vi "FunctDataMgr.Update Meas Data.vi"(8 "error in (no error)":errorcluster, 10 "Data.Meas":T1[](array[typedef]) {"Status" items=["LOG", "PASS", "FAIL", "ERROR"]}, 11 "FunctDataMgr in":refnum<class "FunctDataMgr.lvclass">) -> (0 "error out":errorcluster, 3 "FunctDataMgr out":refnum<class "FunctDataMgr.lvclass">)   [LabVIEW 2024, in "FunctDataMgr.lvclass"]
uses:
  FunctDataMgr.lvclass
  Results/Result.Measurement Item.ctl
  Results/Result.Measurement and Attribute Item Status.ctl
  FunctDataMgr.lvclass/FunctDataMgr.ctl
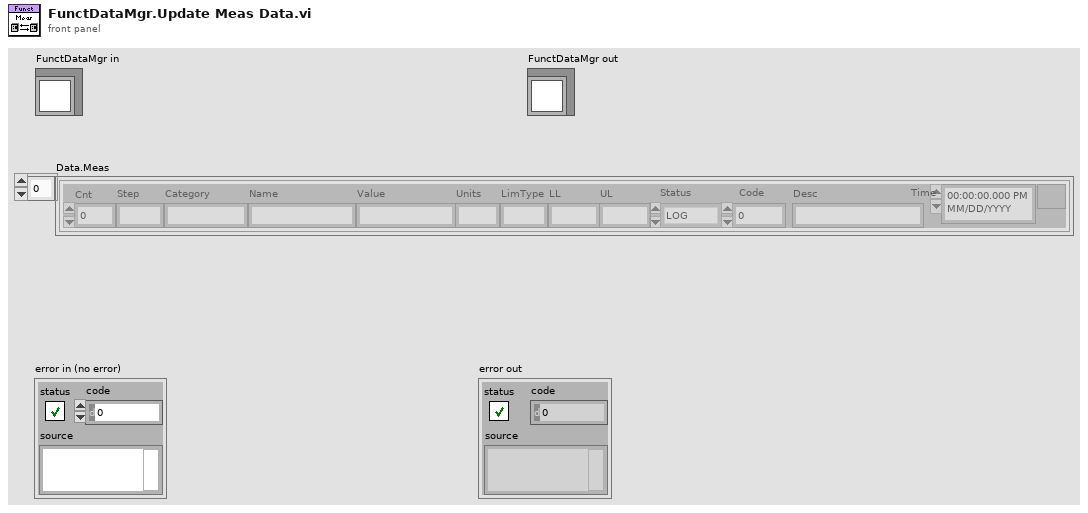
[diagram p1: front panel]
types:
  T1 = typedef "Result.Measurement Item.ctl" = cluster{"Cnt":i32, "Step":string, "Category":string, "Name":string, "Value":string, "Units":string, "LimType":string, "LL":string, "UL":string, "Status":T2, "Code":i32, "Desc":string, "Time":timestamp}
  T2 = typedef "Result.Measurement and Attribute Item Status.ctl" = i32
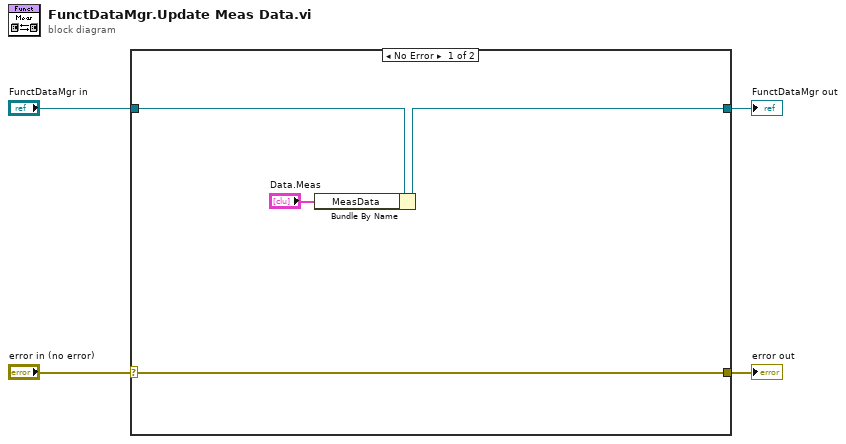
[diagram p0: block diagram]
diagram:
  n1 = case shown="No Error" "error in (no error)" {
    selector: "error in (no error)" -> [w8 w10]
    tunnel: [w8 w10] -> w3
    tunnel: [w6 w9] -> w1
    tunnel: "FunctDataMgr in" -> [w7 w9]
    frame No Error {
      n2 = Bundle By Name(cluster=w7, "MeasData"="Data.Meas") -> (w6:refnum<class "FunctDataMgr.lvclass">)
    }
    frame Error {
    }
  }
  "error out" <- w3
  "FunctDataMgr out" <- w1
